vi "setup Output Pin Msk LV.vi"(10 "OutputPinMsk":u16, 11 "instance":i32) -> (3 "function return":u32)   [LabVIEW 2025, in "SADI_FW3.lvlib"]
doc: "SADI_API_Wrapper unsigned int setupOutputPinMsk_LV( int instance,uint16_t OutputPinMsk );"
uses:
  SADI_FW3.lvlib
  SADI_FW3.dll
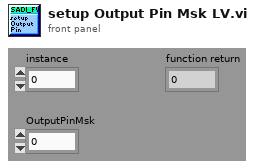
[diagram p1: front panel]
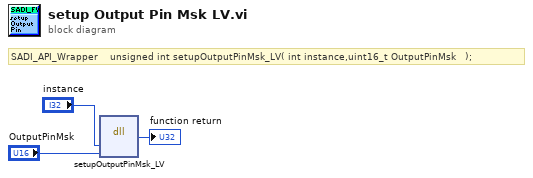
[diagram p0: block diagram]
diagram:
  # "SADI_API_Wrapper    unsigned int setupOutputPinMsk_LV( int instance,uint16_t OutputPinMsk   );"
  n1 = dll-call lib="C:/Users/noaht/iCloudDrive/#1 School/Fall 2025/Controls Lab/LabView/EML4314c_FA25_framework_0/LVLib/SADI_FW3.*" fn="setupOutputPinMsk_LV"("instance"="instance", "OutputPinMsk"="OutputPinMsk") -> (→"function return":u32)  [unwired: 5 in, 2 out]
